vi "Calculate CRC16_CCITT(0x1024).vi"(9 "CRC Init Value(0x0000)":u16 format="%04x", 11 "Data in":u8[](array[numeric]) format="%02x") -> (0 "Lo CRC16":u8 format="%02x", 1 "Hi CRC16":u8 format="%02x", 2 "CRC16_CCITT":u16 format="%.0x", 3 "Data out":u8[](array[numeric]) format="%02x")   [LabVIEW 2013]
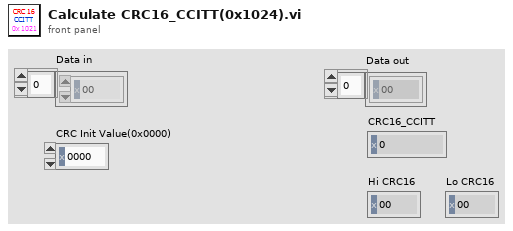
[diagram p1: front panel]
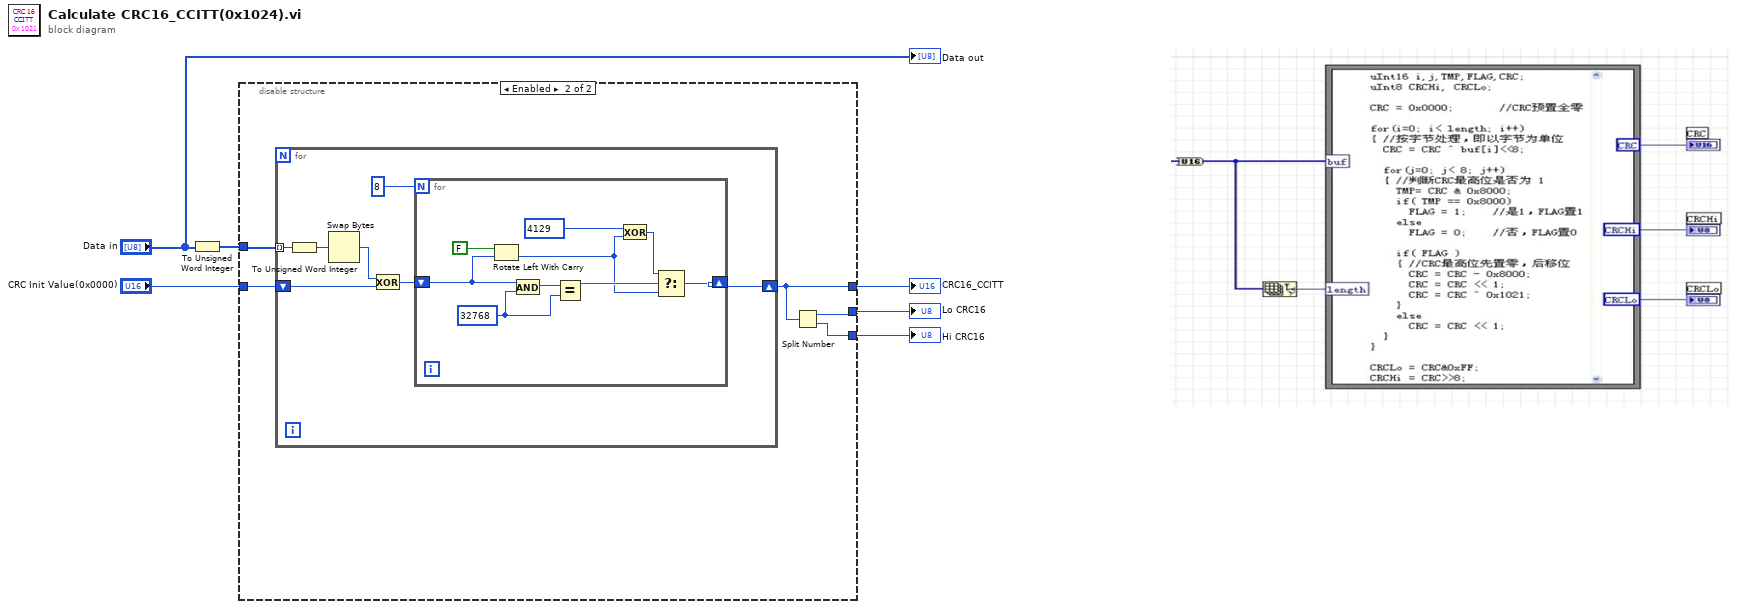
[diagram p0: block diagram]
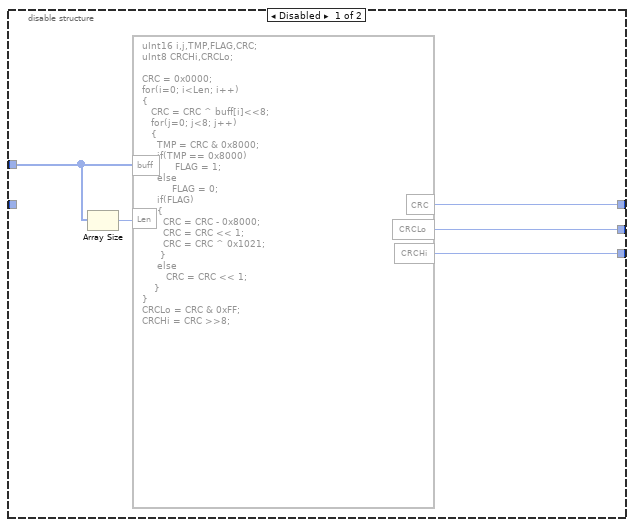
[diagram p2: hidden frame]
diagram:
  n1 = To Unsigned Word Integer(number="Data in") -> (unsigned 16bit integer=w3:u16[])
  n2 = disable-structure shown="Enabled" {
    disable-tunnel: [w11 w14] -> w6
    disable-tunnel: w3 -> [w10 w16]
    disable-tunnel: [w8 w13] -> w5
    disable-tunnel: [w7 w12] -> w4
    disable-tunnel: "CRC Init Value(0x0000)" -> [_ w15]
    frame Disabled {
      n3 = Array Size(array=w10) -> (size(s)=w9:i32)
      n4 = formula code="uInt16 i,j,TMP,FLAG,CRC;\nuInt8 CRCHi,CRCLo;\n\nCRC = 0x0000;\nfor(i=0; i<Len; i++)\n{\n   CRC = CRC ^ buff[i]<<8;\n   for(j=0; j<8; j++)\n   {\n     TMP = CRC & 0x8000;\n     if(TMP == 0x8000)\n           FLAG = 1;\n     else\n          FLAG = 0;\n     if(FLAG)\n     {\n       CRC = CRC - 0x8000;\n       CRC = CRC << 1;\n       CRC = CRC ^ 0x1021;\n      }\n     else\n        CRC = CRC << 1;\n    }\n}\nCRCLo = CRC & 0xFF;\nCRCHi = CRC >>8;"("buff"=w10, "Len"=w9) -> ("CRC"=w11:u16, "CRCLo"=w8:u8, "CRCHi"=w7:u8)
    }
    frame Enabled {
      n5 = for {
        tunnel: w16 -> [w23] mode=indexing
        shift-right: [w17] -> w14
        shift-left: w15 -> [w20]
        n6 = To Unsigned Word Integer(number=w23) -> (unsigned 16bit integer=w22:u16)
        n7 = Swap Bytes(anything=w22) -> (byte swapped=w21:u16)
        n8 = Exclusive Or(1:w20, 2:w21) -> (0:w19:u16)
        n9 = for {
          N: 8 -> [_]
          shift-right: [w24] -> w17
          shift-left: w19 -> [w29]
          w31 = u16 32768 ("y")
          n10 = Rotate Left With Carry(2:w29, 3:FALSE ("carry")) -> (0:w27:u16)  [unwired: 1 out]
          n11 = And(x=w29, y=w31) -> (x .and. y?=w32:u16)
          n12 = Equal?(x=w32, y=w31) -> (x = y?=w30:bool)
          n13 = Exclusive Or(1:w27, 2:u16 4129 ("y")) -> (0:w25:u16)
          n14 = Select(t=w25, s=w30, f=w27) -> (s? t:f=w24:u16)
        }
      }
      n15 = Split Number(x=w14) -> (hi(x)=w13:u8, lo(x)=w12:u8)
    }
  }
  "Lo CRC16" <- w5
  "Hi CRC16" <- w4
  "CRC16_CCITT" <- w6
  "Data out" <- "Data in"
